vi "Create.vi"(8 "error in (no error)":errorcluster, 9 "Node":string, 10 "MsgQ":refnum<class "MessageQ.lvclass">) -> (0 "error out":errorcluster, 3 "VectoEventBridge out":refnum<class "VectoEventBridge.lvclass">)   [LabVIEW 2020, in "Volatus.lvlib" / "VectoEventBridge.lvclass"]
uses:
  VectoEventBridge.lvclass
  MessageQ/MessageQ.lvclass
  VectoEventBridge.lvclass/VectoEventBridge.ctl
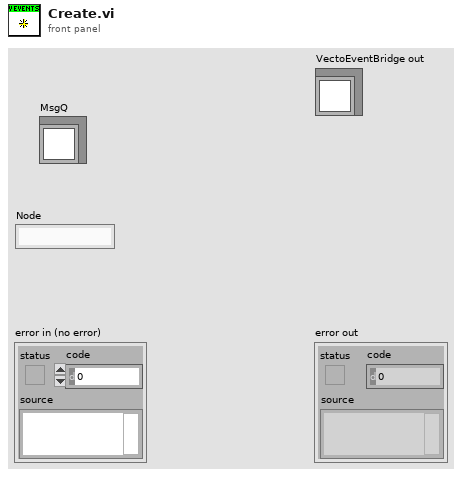
[diagram p1: front panel]
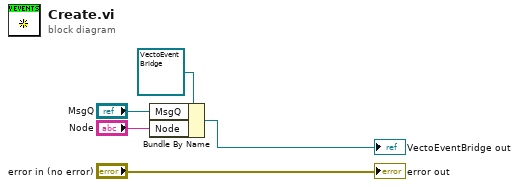
[diagram p0: block diagram]
diagram:
  n1 = Bundle By Name(cluster=refnum<class "VectoEventBridge.lvclass"> refnum ("VectoEventBridge in"), "MsgQ"="MsgQ", "Node"="Node") -> (→"VectoEventBridge out":refnum<class "VectoEventBridge.lvclass">)
  "error out" <- "error in (no error)"
